vi "Digitizer Analyze_Phase Noise.vi"(6 "band":T1 {"stop frequency (Hz)" format="%.2f"; "start frequency (Hz)" format="%.2f"}, 7 "Pins":string[](array[string])=["Xout"], 9 "Published Data Id":string[](array[string]), 10 "Waveform Data In":waveform(dbl)[](array[waveform])=[{"t0"=timestamp(3637030365.2340937 s since 1904-01-01), "dt"=3.3333333333333334e-08, "Y"=array[5343 elements]}, {"t0"=timestamp(3637030365.2340937 s since 1904-01-01), "dt"=3.3333333333333334e-08, "Y"=array[5343 elements]}], 11 "Semiconductor Module Context":T2) -> (0 "error out":errorcluster, 3 "Phase Noise (dBm)":dbl[](array[numeric]))   [LabVIEW 2014]
doc: "Example: Measurement Library\n\nRecommended Input Signal: 100 kHz, 2 Vpp, sine wave\n\nDevices Supported: Refer to NI Example Finders\n\nLabVIEW Description:\n\nThis example illustrates fetching scalar measurements from NI-SCOPE, such as period and rise time calculations. \n\nSome common horizontal and vertical parameters are configured for the oscilloscope. The property node is used to set the reference level units, and the low, middle and high reference levels. For more information about measurement library parameters, see the NI-SCOPE VI Reference Help file. \n\nAfter the Read VI is called to acquire a waveform, the Fetch Measurement Stats VI is used to perform the desired scalar measurement analysis on the waveform. NI-SCOPE keeps a history of each measurement's results, which allows it to retrieve the statistics computed over multiple acquisitions. These statistics include the mean, standard deviation, min, max and number of acquisitions used in the statistics. The statistics are updated once per acquisition when the measurement is fetched. The Clear Stats VI clears this history."
uses:
  <vilib>/NI_TestStand_SemiconductorModule/NI_TestStand_Semiconductor_Module.lvlibp/PinMap/General/SemiconductorModuleContext.ctl
  <vilib>/NI_TestStand_SemiconductorModule/NI_TestStand_Semiconductor_Module.lvlibp/PinMap/General/NIInstrumentTypeIDs.ctl
  <vilib>/addons/jitter/shared/controls/ja_time axis.ctl
  <vilib>/NI_TestStand_SemiconductorModule/NI_TestStand_Semiconductor_Module.lvlibp/PinMap/General/Publish/PublishDataDoubleFunctionalTest.vi
  <vilib>/NI_TestStand_SemiconductorModule/NI_TestStand_Semiconductor_Module.lvlibp
  <vilib>/addons/jitter/NI_JAT.lvlib
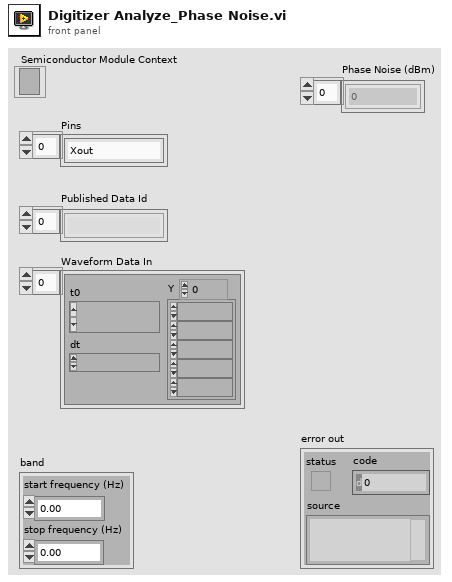
[diagram p1: front panel]
types:
  T1 = cluster{"start frequency (Hz)":dbl, "stop frequency (Hz)":dbl}
  T2 = typedef "NI_TestStand_Semiconductor_Module.lvlibp/SemiconductorModuleContext.ctl" = refnum<k7>
  T3 = typedef "NI_TestStand_Semiconductor_Module.lvlibp/NIInstrumentTypeIDs.ctl" = string
  T4 = typedef "NI_JAT.lvlib/ja_time axis.ctl" = cluster{"indexes":dbl[], "t0":timestamp, "dt":dbl}
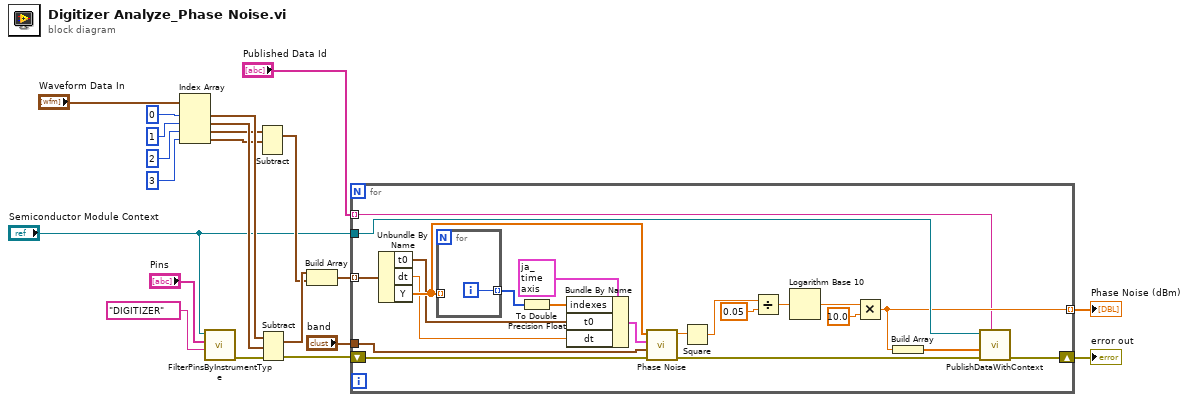
[diagram p0: block diagram]
diagram:
  n1 = Index Array(array="Waveform Data In", index #1=0 ("index"), index #2=1 ("index"), index #3=2 ("index"), index #4=3 ("index")) -> (element #1=w14:waveform(dbl), element #2=w13:waveform(dbl), element #3=w8:waveform(dbl), element #4=w7:waveform(dbl))
  n2 = call <vilib>:"FilterPinsByInstrumentType.vi"("Instrument Type Id"=T3 "DIGITIZER", "Pins"="Pins", "Semiconductor Module Context"="Semiconductor Module Context") -> ("error out"=w12:errorcluster)  [unwired: 6 in, 2 out]
  n3 = Subtract(1:w7, 2:w8) -> (0:w6:waveform(dbl))  [unwired: 1 in, 1 out]
  n4 = Subtract(1:w13, 2:w14, 4:w12) -> (0:w9:waveform(dbl), 3:w15:errorcluster)
  n5 = Build Array(w9, w6) -> (w5:waveform(dbl)[])
  n6 = for {
    tunnel: "band" -> [w43]
    tunnel: w5 -> [w42] mode=indexing
    tunnel: [w24] -> w4 mode=indexing
    shift-right: [w26] -> w3
    shift-left: w15 -> [w28]
    tunnel: "Semiconductor Module Context" -> [w25]
    tunnel: "Published Data Id" -> [w22] mode=indexing
    n7 = Unbundle By Name(w42) -> ("t0"=w39:timestamp, "dt"=w38:dbl, "Y"=w41:dbl[])
    n8 = for {
      tunnel: w41 -> [_] mode=indexing
      tunnel: [w44] -> w37 mode=indexing
      i -> [w44]
    }
    n9 = To Double Precision Float(number=w37) -> (double precision float=w36:dbl[])
    n10 = Bundle By Name(cluster=T4 {"indexes"=[], "t0"=timestamp(0 s since 1904-01-01), "dt"=0.0} ("jitter timestamps"), "indexes"=w36, "t0"=w39, "dt"=w38) -> (w35:T4)
    n11 = call <vilib>:"Phase Noise.vi"("error in"=w28, "band"=w43, "jitter timestamps"=w35, "jitter sequence"=w41) -> ("error out"=w27:errorcluster, "phase noise in band (s rms)"=w32:dbl)  [unwired: 5 in, 1 out]
    n12 = Square(x=w32) -> (x^2=w31:dbl)
    n13 = Divide(x=w31, y=0.05) -> (x/y=w29:dbl)
    n14 = Logarithm Base 10(1:w29) -> (0:w34:dbl)
    n15 = Multiply(x=w34, y=10.0) -> (x*y=w24:dbl)
    n16 = Build Array(w24) -> (w23:dbl[])
    n17 = call-poly <vilib>:"PublishDataWithContext.vi"("Published Data Id"=w22, "error in (no error)"=w27, "Data In"=w23, "Semiconductor Module Context"=w25) -> ("error out"=w26:errorcluster)  [unwired: 6 in, 1 out]
  }
  "error out" <- w3
  "Phase Noise (dBm)" <- w4
